vi "ep_Check Stator Resistance.vi"(8 "error in (no error)":errorcluster, 11 "stator resistance  [ohms]":dbl) -> (0 "error out":errorcluster)   [LabVIEW 2014, in "NI_EP_Motor Monitoring.lvlib"]
uses:
  <vilib>/addons/Electrical Power/Motor Monitoring/NI_EP_Motor Monitoring.lvlib
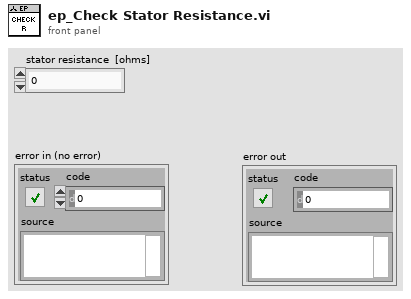
[diagram p1: front panel]
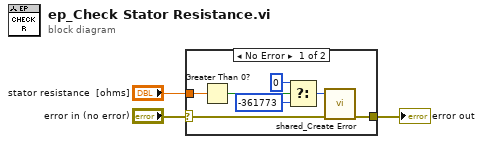
[diagram p0: block diagram]
diagram:
  n1 = case shown="No Error" "error in (no error)" {
    selector: "error in (no error)" -> [w8 w11]
    tunnel: [w7 w11] -> w2
    tunnel: "stator resistance  [ohms]" -> [w5 _]
    frame No Error {
      n2 = Greater Than 0?(x=w5) -> (x > 0?=w4:bool)
      n3 = Select(t=0, s=w4, f=-361773 ("error code (0)")) -> (s? t:f=w6:i32)
      n4 = call <vilib>:"shared_Create Error.vi"("error in (no error)"=w8, "error code (0)"=w6) -> ("error out"=w7:errorcluster)  [unwired: 9 in]
    }
    frame Error {
    }
  }
  "error out" <- w2
